vi "Kinesis - KDC101 - Get Position.vi"() -> ()   [LabVIEW 2012]
uses:
  U:/Kinesis LabVIEW Website Examples/Thorlabs.MotionControl.Controls.dll
  Thorlabs.MotionControl.Controls.dll
  U:/Kinesis LabVIEW Website Examples/ThorLabs.MotionControl.KCube.DCServoCLI.dll
  ThorLabs.MotionControl.KCube.DCServoCLI.dll
panel:
  in  "Stop":bool
  out "Position (mm)":i32
  in  "SerialNumber":string
  in  "KCubeDCServoControl":refnum<k24>(container)
  # "Notes:"
  # "- Ensure that the appropriate .DLLs are copied into your Project Folder. Check that the correct bit type are used depending on your version of LabVIEW\ni.e. 32-bit or 64-bit.\n\n\n\n\n\n\n\n\n\n\n\n\n\n- Open the example VI through the LabVIEW Project Explorer to correctly load the User Interface from Thorlabs.MotionControl.Controls.dll."
  # "Thorlabs Hardware: KDC101 - K-Cube Brushed DC Servo Motor Controller\nhttps://www.thorlabs.com/newgrouppage9.cfm?objectgroup_id=2419&pn=KDC101#5077\n\n\nDescription: This VI shows how to poll the device position outside of the device UI. The function GetPositionCounter() will output the stage position in Device Units. This can be converted from Device Units (Encoder Counts) to Real World Units (mm) by considering Encdoer Counts per revolution of the motor, Gearbox Ratios & Leadscrew Pitch. Details of this calculation are highlighted in the VI.\n\nInstructions:\n1) Connect your KDC101 device to your PC & power the device, ensuring your stage/actutator is connected. \nFor full device setup, the device product manual can be found on our website here. - https://www.thorlabs.com/thorproduct.cfm?partnumber=KDC101\n2) Enter the device serial number below.\n3) Click 'Run' in the LabVIEW Toolbar.\n4) To end the program, click 'STOP'."
  # "Example Image of .NET Controller - VI opened via Project Explorer/ not opened via Project Explorer"
  # "VI Not Opened via Project Explorer"
  # "VI Opened via Project Explorer"
  # "How to Calculate the Linear Displacement per Encoder Count\n\nFor the Z812 and Z812B, there are 512 encoder counts per revolution of the motor. The output shaft of the motor goes into a 67:1 planetary gear head. This requires the motor to rotate 67 times to rotate the 1.0 mm pitch lead screw one revolution. The end result is the lead screw advances by 1.0 mm. The linear displacement of the actuator per encoder count is given by\n\n512 x 67 = 34,304 encoder counts per revolution of the lead screw,\n\nwhereas the linear displacement of the lead screw per encoder count is given by\n\n1.0 mm / 34,304 counts = 2.9 x 10-5 mm (29 nm)."
  # "- To explore the range of methods available, please visit the .NET API, included with your Kinesis software.\n- For tips on building your own VIs with Thorlabs Motion Control Hardware, please see our LabVIEW Guide here.\nhttps://www.thorlabs.com/newgrouppage9.cfm?objectgroup_id=10285"
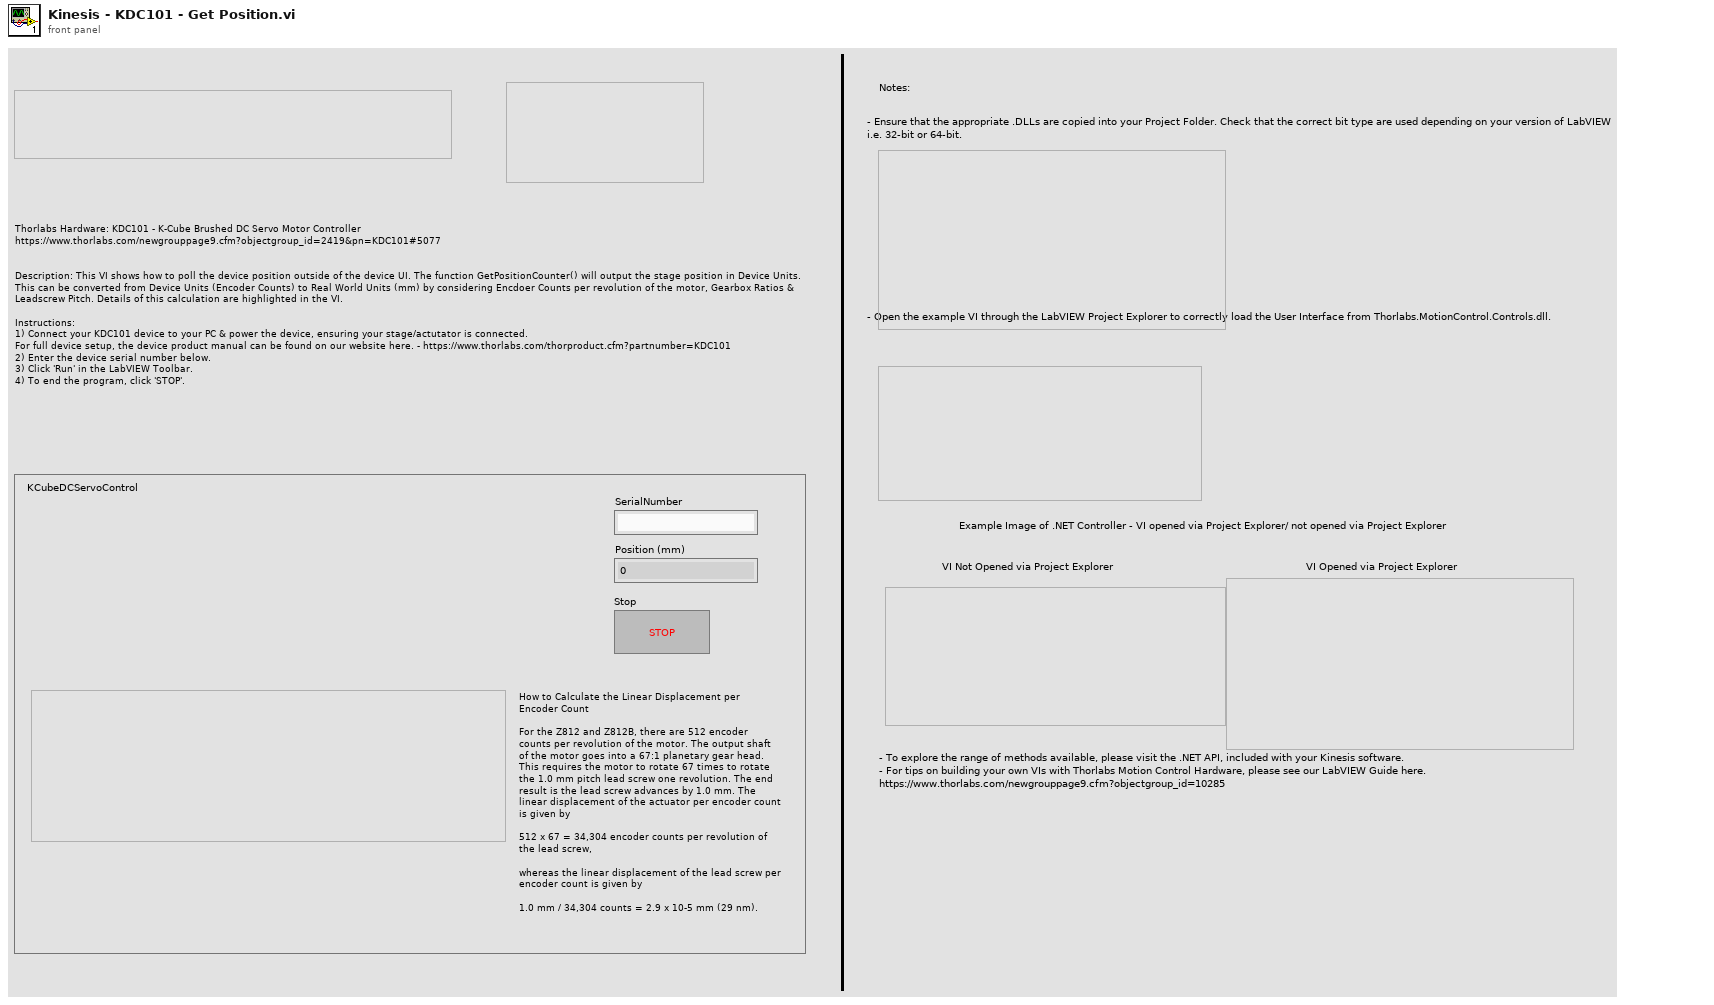
[diagram p1: front panel]
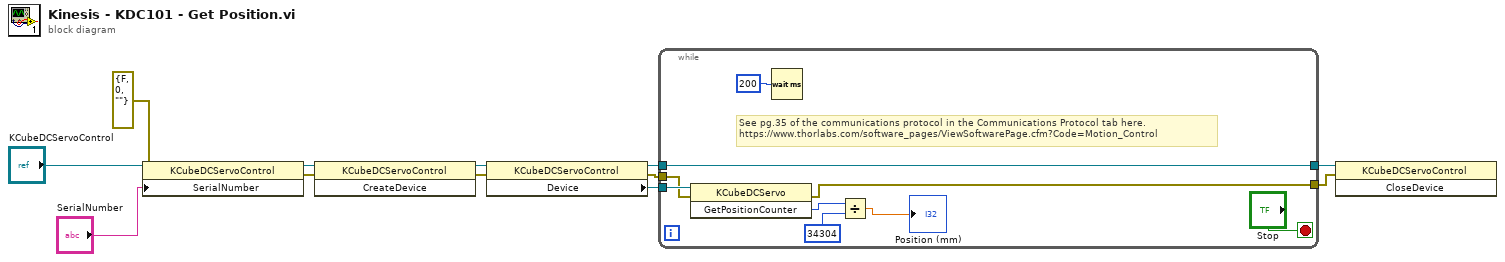
[diagram p0: block diagram]
diagram:
  n1 = property class="KCubeDCServoControl"(reference="KCubeDCServoControl", error in=errorcluster {"status"=FALSE, "code"=0, "source"=""} ("error in (no error)"), "SerialNumber"="SerialNumber") -> (reference out=w10:refnum<k24>, error out=w6:errorcluster)
  n2 = invoke class="KCubeDCServoControl" method="CreateDevice"(reference=w10, error in=w6) -> (reference out=w9:refnum<k24>, error out=w5:errorcluster)  [unwired: 1 in, 1 out]
  n3 = property class="KCubeDCServoControl"(reference=w9, error in=w5) -> (reference out=w7:refnum<k24>, error out=w3:errorcluster, "Device"=w4:refnum<k24>)
  n4 = while {
    tunnel: w4 -> [w21]
    tunnel: [w20] -> w8
    tunnel: w7 -> [w20]
    tunnel: w3 -> [w14]
    tunnel: [w13] -> w2
    stop <- "Stop" stop-if-true
    # "See pg.35 of the communications protocol in the Communications Protocol tab here.\nhttps://www.thorlabs.com/software_pages/ViewSoftwarePage.cfm?Code=Motion_Control"
    n5 = invoke class="KCubeDCServo" method="GetPositionCounter"(reference=w21, error in=w14) -> (error out=w13:errorcluster, "GetPositionCounter"=w16:i32)  [unwired: 1 in, 1 out]
    n6 = Wait (ms)(milliseconds to wait=u32 200) -> ()  [unwired: 1 out]
    n7 = Divide(x=w16, y=34304 ("GetPositionCounter")) -> (x/y=→"Position (mm)":dbl)
  }
  n8 = invoke class="KCubeDCServoControl" method="CloseDevice"(reference=w8, error in=w2) -> ()  [unwired: 1 in, 3 out]
